vi "08a_Fronta Zaklady.vi"() -> ()   [LabVIEW 2012]
doc: "Tento příklad demonstruje plnění fronty daty různou rychlostí a chování pří zaplnění fronty. Blokový diagram obsahuje jednu smyčku, která plní frontu daty a druhou, která data vyčítá. U obou smyček lze volit rychlosti jejich běhu.\n\nPokud je rychlost vkládání dat do fronty menší než rychlost vyčítání, počet prvků ve frontě klesá. Po vyprázdnění fronty se rychlost smyčky provádějící vyčítání se synchronizuje s rychlostí vkládání (čeká na nové data).\n\nPokud je rychlost vkládání dat do fronty větší než rychlost vyčítání, počet prvků ve frontě roste. Po zaplnění fronty se rychlost smyčky provádějící vkládání dat se synchronizuje s rychlostí vyčítání (čeká na místo ve frontě)."
panel:
  out "Poslední Vyčtený Prvek":dbl format="%0.2f"
  in  "Rychlost Vkládání":bool
  in  "Rychlost Vyčítání":bool
  out "Graf":cluster{"Last Element Inserted":dbl, dbl}(graph)
  out "Prvků ve Frontě":i32(slide) scale=0.0..50.0 scale format="%0.0f"
  in  "stop":bool
  in  "Velikost Fronty":i32=50
  out "Poslední Vložený Prvek":dbl format="%0.2f"
  # "Použití:\n1. Nastavit velikost fronty.\n2. Spusti VI.\n3. Měnit rychlost vkládání a vyčítání dat."
  # "100 ms\n\n500 ms"
  # "100 ms\n\n500 ms"
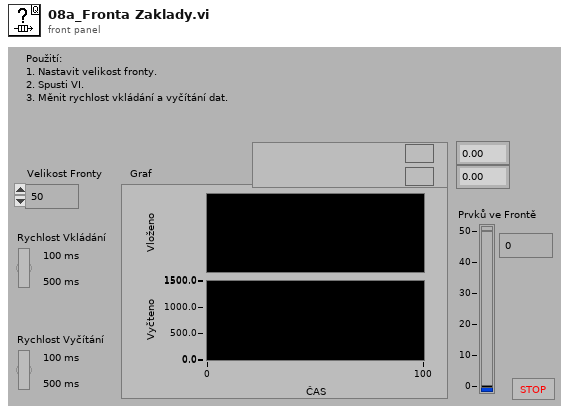
[diagram p1: front panel]
types:
  T1 = cluster{"Poslední Vložený Prvek":dbl, "Poslední Vyčtený Prvek":dbl}
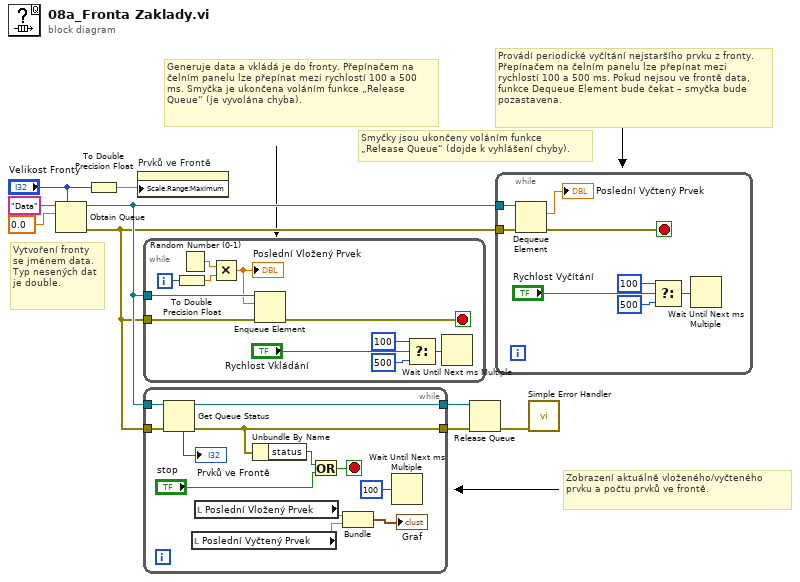
[diagram p0: block diagram]
diagram:
  # "Smyčky jsou ukončeny voláním funkce \n„Release Queue“ (dojde k vyhlášení chyby)."
  # "Provádí periodické vyčítání nejstaršího prvku z fronty. Přepínačem na čelním panelu lze přepínat mezi rychlostí 100 a 500 ms. Pokud nejsou ve frontě data, funkce Dequeue Element bude čekat – smyčka bude pozastavena."
  # "Zobrazení aktuálně vloženého/vyčteného \nprvku a počtu prvků ve frontě."
  # "Generuje data a vkládá je do fronty. Přepínačem na čelním panelu lze přepínat mezi rychlostí 100 a 500 ms. Smyčka je ukončena voláním funkce „Release Queue“ (je vyvolána chyba)."
  # "Vytvoření fronty se jménem data.\nTyp nesených dat je double."
  n1 = Obtain Queue(max queue size (-1, unlimited)="Velikost Fronty", name (unnamed)="Data", element data type=0.0) -> (queue out=w9:refnum<queue>, error out=w4:errorcluster)  [unwired: 2 in, 1 out]
  n2 = To Double Precision Float(number="Velikost Fronty") -> (double precision float=w8:dbl)
  n3 = property on="Prvků ve Frontě" class="Slide (strict)"("Scale.Range:Maximum"=w8) -> ()  [unwired: 2 in, 2 out]
  n4 = while {
    tunnel: w9 -> [w20]
    tunnel: w4 -> [w11]
    i -> [w18]
    stop <- w10 stop-if-true
    n5 = To Double Precision Float(number=w18) -> (double precision float=w17:dbl)
    n6 = Random Number (0-1)() -> (number: 0 to 1=w19:dbl)
    n7 = Multiply(x=w19, y=w17) -> (x*y=w16:dbl)
    "Poslední Vložený Prvek" <- w16
    n8 = Enqueue Element(queue=w20, element=w16, error in (no error)=w11) -> (error out=w10:errorcluster)  [unwired: 3 out]
    n9 = Select(t=u32 100, s="Rychlost Vkládání", f=u32 500) -> (s? t:f=w12:u32)
    n10 = Wait Until Next ms Multiple(millisecond multiple=w12) -> ()  [unwired: 1 out]
  }
  n11 = while {
    tunnel: w9 -> [w32]
    tunnel: [w21] -> w3
    tunnel: w4 -> [w25]
    tunnel: [w22] -> w2
    stop <- w28 stop-if-true
    n12 = Get Queue Status(queue=w32, error in (no error)=w25) -> (queue out=w22:refnum<queue>, error out=w21:errorcluster, # elements in queue=→"Prvků ve Frontě":i32)  [unwired: 6 out]
    n13 = local read "Poslední Vyčtený Prvek"() -> (w23:dbl)
    n14 = local read "Poslední Vložený Prvek"() -> (w24:dbl)
    n15 = Unbundle By Name(w21) -> ("status"=w27:bool)
    n16 = Or(x=w27, y="stop") -> (x .or. y?=w28:bool)
    n17 = Bundle("Poslední Vložený Prvek"=w24, "Poslední Vyčtený Prvek"=w23) -> (→"Graf":T1)  [unwired: 1 out]
    n18 = Wait Until Next ms Multiple(millisecond multiple=u32 100 ("milliseconds to wait")) -> ()  [unwired: 1 out]
  }
  n19 = Release Queue(queue=w2, error in (no error)=w3) -> (error out=w1:errorcluster)  [unwired: 3 out]
  n20 = while {
    tunnel: w9 -> [w40]
    tunnel: w4 -> [w34]
    stop <- w33 stop-if-true
    n21 = Dequeue Element(queue=w40, error in (no error)=w34) -> (element=→"Poslední Vyčtený Prvek":dbl, error out=w33:errorcluster)  [unwired: 3 out]
    n22 = Select(t=u32 100, s="Rychlost Vyčítání", f=u32 500) -> (s? t:f=w36:u32)
    n23 = Wait Until Next ms Multiple(millisecond multiple=w36) -> ()  [unwired: 1 out]
  }
  n24 = call <vilib>:"Simple Error Handler.vi"("error in (no error)"=w1) -> ()  [unwired: 1 in, 8 out]
